vi "NF87XX.get motor type.vi"(0 "i ref in":refnum<vi>, 2 "System":string="N/A", 3 "Motor (0, 1, 2)":i32, 5 "error in (no error)":errorcluster) -> (14 "i ref out":refnum<vi>, 16 "Motor Type":T2=enum."not defined", 19 "error out":errorcluster)   [LabVIEW 2014, in "NF87XX.lvlib"]
doc: "Returns the configured motor type which is either \"0\" (standard picomotor) or \"1\" (tiny picomotor). The connected motor may be another type and has to be configured right in this case.\n\nauthor: Stefan Götte\ndata: 09-JAN-2007\n\n\nLicense Agreement for this software:\n\nCopyright (C)\nGesellschaft für Schwerionenforschung, GSI\nPlanckstr. 1\n64291 Darmstadt\nGermany\n\nContact: D.Beck@gsi.de \n\nThis program is free software; you can redistribute it and/or modify it under the terms of the GNU General Public License as published by the Free Software Foundation; either version 2 of the license, or (at your option) any later version.\n\nThis program is distributed in the hope that it will be useful, but WITHOUT ANY WARRANTY; without even the implied warranty of MERCHANTABILITY or FITNESS FOR A PARTICULAR PURPOSE. See the GNU General License for more details (http://www.gnu.org).\n\nGesellschaft für Schwerionenforschung, GSI\nPlanckstr. 1, 64291 Darmstadt, Germany\nFor all questions and ideas contact: M.Richter@gsi.de, H.Brand@gsi.de or D.Beck@gsi.de.\nLast update: 17-JUN-2004"
uses:
  NF87XX.lvlib
  NF87XX.motor Type.ctl
  non_GPL/instr.lib/NewFocusPico/Pico Parameters.ctl
  CSCore/CSSystem/CoreDefs/CoreDefs.error_type.ctl
  CSCore/CSSystem/CoreLib/CoreLib.lvlib
  non_GPL/instr.lib/NewFocusPico/NewFocusPico - Driver np.lvlib
panel:
  in  "Pico Parameter":T1={"Pico Type"=enum."Open-Loop Pico", "Acceleration (steps/sec^2)"="32000", "Velocity ( Hz)"="2000", "Driver"="A1", "Motor"="0", "Channel"="0", "Process Step"="Final Test"}
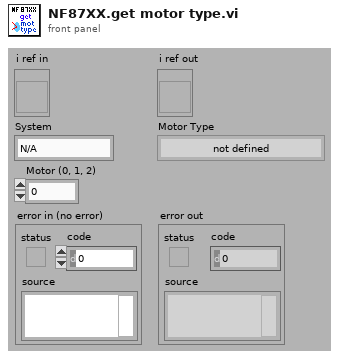
[diagram p1: front panel]
types:
  T1 = typedef "NewFocusPico - Driver np.lvlib/Pico Parameters.ctl" = cluster{"Pico Type":enum16{"Open-Loop Pico", "Close-Loop Pico", "Pico Ultra"}, "Acceleration (steps/sec^2)":string, "Velocity ( Hz)":string, "Driver":string, "Motor":string, "Channel":string, "Process Step":string}
  T2 = typedef "NF87XX.lvlib/NF87XX.motor Type.ctl" = enum16{"Standard Picomotor", "Tiny Picomotor", "not defined"}
  T3 = typedef "CoreDefs.error_type.ctl" = enum16{"no error", "can't load process", "can't unload process", "process does not exist", "can't install process", "can't remove process", "unknown function", "time out", "can't execute function", "duplicate queue name", "super not found", "caller queue invalid", "can't ping process", "unknown error", "VISA Error", "VISA timeout", "GPIB timeout", "GPIB error", "communication error", "data type mismatch", "can't read data from OPC server", "can't write data to OPC server", "OET error", "function not implemented", "process already exists", "invalid Shared Variable name", "error writing Shared Variable", "error reading Shared Variable", "invalid client name", "corrupt database", "unknown class", "call not authorized", "parameter out of range", "OET timeout: can't get data to modify", "invalid queue name", "requested operation incompatible with current state", "event undefined", "event disabled", "state undefined", "caller is not a friend", "EventBuilder: bad eventID", "EventBuilder: no DAQ devices", "a thread must not stop itself", "UNUSED ELEMENT4", "DiscArchiver: eventData incomplete", "DiscArchiver: eventData does not belong to run", "DiscArchiver: can't open file", "DiscArchiver: can't write to file", "DiscArchiver: available disc space low", "can't acquire semaphore", "error reading data from database", "notifier object is not existing", "can't register process", "can't unregister process", "illegal event type", "object disabled", "object already exists", "can't change state", "Instrument not found", "no connection to remote node", "invalid reference", "N/A", "UNUSED ELEMENT 1", "element not found", "illegal TCP/IP connection detected", "object does not exist", "invalid access ID", "unknown CS system", "invalid privilige", "unsupported data type", "unsupported server type", "IO server already exists", "Shared Variable already exists"}
  T4 = enum16{"User....", "DEF", "DIAG", "INI", "LOCK", "UNLOCK", "MAP", "SAV", "VER", "ACC", "CHL", "FOR", "GO", "HAL", "MOF", "MON", "MPV", "POS", "REL", "REV", "STA", "STO", "TYP", "VEL", "ABS", "SER", "NOS", "DRT", "FLI", "RLI", "FIN", "RIN", "AIN", "IN", "JOF", "JON", "OUT", "RES FINE", "RES COARSE", "02 (HEX)", "PWM", "CNT", "TMR", "HOSTNAME", "IPADDR", "IPMODE", "NETMASK", "GATEWAY", "DNSSRVR", "PASSWD", "ECHO", "MACADDR"}
  T5 = typedef "NF87XX.lvlib/NF87XX.driver Type.ctl" = enum16{"not defined", "3-ch open loop drv", "1-ch closed loop drv"}
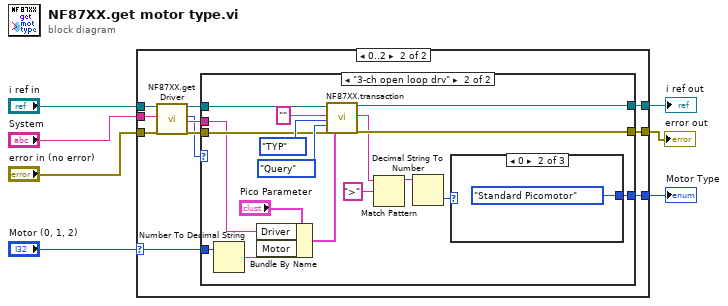
[diagram p0: block diagram]
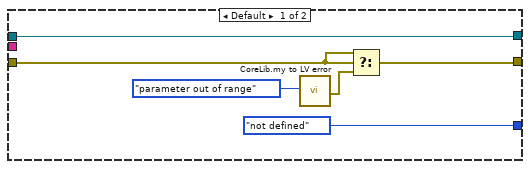
[diagram p2: hidden frame]
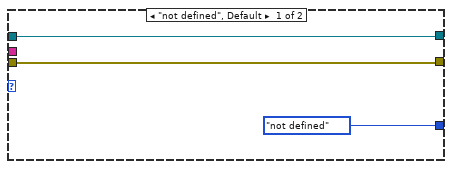
[diagram p3: hidden frame]
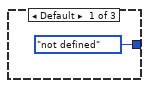
[diagram p4: hidden frame]
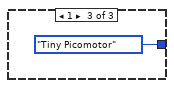
[diagram p5: hidden frame]
diagram:
  n1 = case shown="0..2" "Motor (0, 1, 2)" {
    selector: "Motor (0, 1, 2)" -> [_ w17]
    tunnel: "i ref in" -> [w13 w22]
    tunnel: "error in (no error)" -> [w10 w21]
    tunnel: [w13 w20] -> w5
    tunnel: [w9 w19] -> w4
    tunnel: [NF87XX.motor_Type."not defined" ("Motor Type") w16] -> w3
    tunnel: "System" -> [_ w15]
    frame Default {
      n2 = call "CoreLib.my to LV error.vi"("ErrorTypes"=CoreDefs.error_type."parameter out of range") -> ("myErrorCluster"=w12:errorcluster)  [unwired: 17 in, 1 out]
      n3 = Select(t=w10, s=w10, f=w12) -> (s? t:f=w9:errorcluster)
    }
    frame 0..2 {
      n4 = call "NF87XX.get Driver.vi"("i ref in"=w22, "System"=w15, "error in (no error)"=w21) -> ("i ref out"=w24:refnum<vi>, "Driver Type"=w14:T5, "Driver"=w18:string, "error out"=w23:errorcluster)  [unwired: 12 in, 1 out]
      n5 = case shown="\"3-ch open loop drv\"" w14 {
        tunnel: w24 -> [w27 w42]
        tunnel: w23 -> [w26 w41]
        tunnel: [w27 w39] -> w20
        tunnel: [w26 w38] -> w19
        tunnel: w18 -> [_ w36]
        tunnel: w17 -> [_ w31]
        tunnel: [NF87XX.motor_Type."not defined" ("Motor Type") w29] -> w16
        frame "not defined", Default {
        }
        frame "3-ch open loop drv" {
          n6 = Number To Decimal String(number=w31) -> (decimal integer string=w32:string)  [unwired: 1 in]
          n7 = Bundle By Name(cluster="Pico Parameter", "Driver"=w36, "Motor"=w32) -> (w35:T1)
          n8 = call "NF87XX.transaction.vi"("i ref in"=w42, "User Cmd/Numeric Argu"="", "MCL Cmd"=T4."TYP", "Query/Set"=enum16{"Query", "Set"}."Query", "error in (no error)"=w41, "Pico Parameter"=w35) -> ("i ref out"=w39:refnum<vi>, "Read String"=w33:string, "error out"=w38:errorcluster)  [unwired: 11 in]
          n9 = Match Pattern(string=w33, regular expression=">") -> (before substring=w30:string)  [unwired: 1 in, 3 out]
          n10 = Decimal String To Number(string=w30) -> (number=w28:i32)  [unwired: 2 in, 1 out]
          n11 = case shown="0" w28 {
            tunnel: [NF87XX.motor_Type."not defined" ("Motor Type") NF87XX.motor_Type."Standard Picomotor" ("Motor Type") NF87XX.motor_Type."Tiny Picomotor" ("Motor Type")] -> w29
            frame Default {
            }
            frame 0 {
            }
            frame 1 {
            }
          }
        }
      }
    }
  }
  "error out" <- w4
  "i ref out" <- w5
  "Motor Type" <- w3
